vi "图形化显示数据-1.vi"() -> ()   [LabVIEW 2023]
panel:
  out "Waveform Graph 3":dbl[](graph)
  out "Waveform Chart 3":dbl(graph)
  out "Waveform Graph 2":dbl[](graph)
  out "Waveform Chart 2":dbl(graph)
  out "Waveform Graph":dbl[](graph)
  out "Waveform Chart":dbl(graph)
  # "图形化显示数据"
  # "极坐标系 Polar coordinates 是一种二维坐标系，它使用一个点到原点的距离（称为极径）和该点与正x轴之间的夹角（称为极角）来表示一个点的坐标。"
  # "(r, θ) r 是 极径 点到原点的距离， θ 是 点到 x轴 的 夹脚， 通常 极坐标 用来处理 正数。"
  # "LabVIEW 中最常见的曲线格式是在一个直角坐标系中用 X 轴表示时间，Y 轴表示数据值。"
  # "分析数据走向趋势"
  # "Chart 会保存以前的数据，因为有缓存区， graph 没有缓存区，每次清空"
  # "chart 的属性节点 选择历史，然后双击历史节点属性 选择 改变输出 为输入"
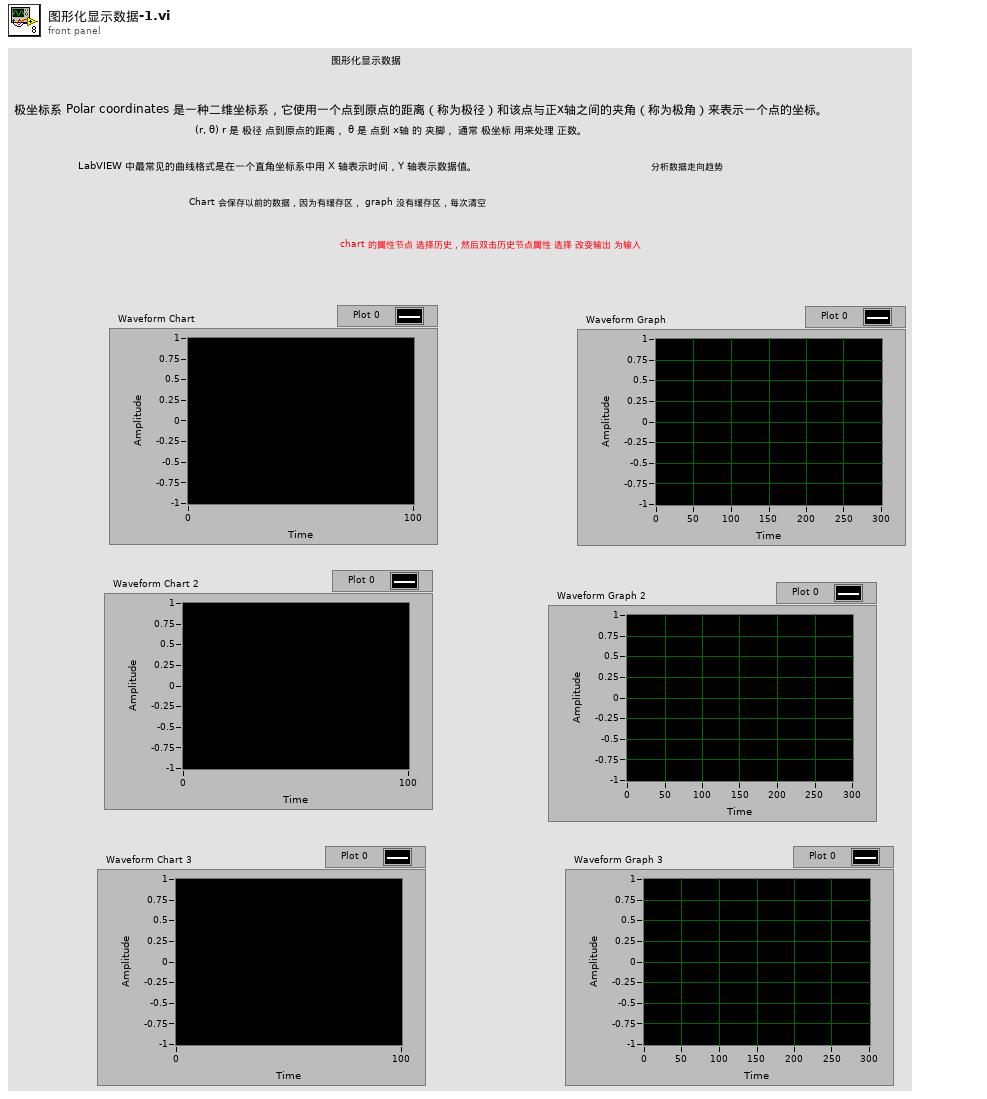
[diagram p1: front panel]
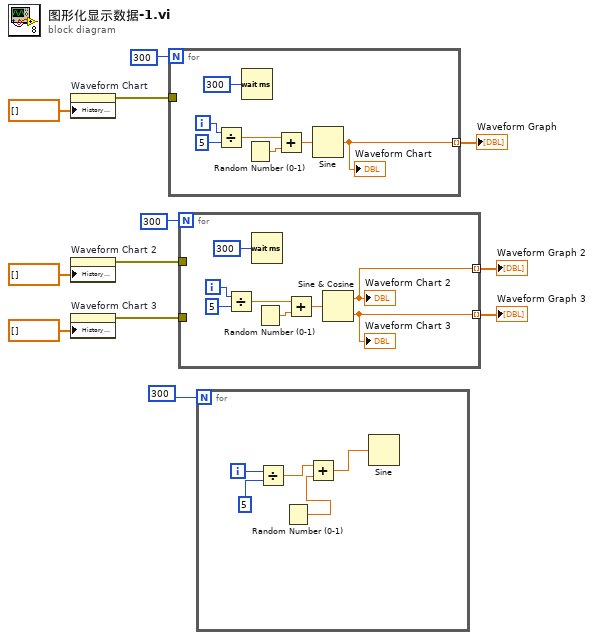
[diagram p0: block diagram]
diagram:
  n1 = property on="Waveform Chart" class="WFChart (strict)"("History Data"=dbl[] []) -> (error out=w6:errorcluster)  [unwired: 2 in, 1 out]
  n2 = property on="Waveform Chart 2" class="WFChart (strict)"("History Data"=dbl[] []) -> (error out=w2:errorcluster)  [unwired: 2 in, 1 out]
  n3 = property on="Waveform Chart 3" class="WFChart (strict)"("History Data"=dbl[] []) -> (error out=w4:errorcluster)  [unwired: 2 in, 1 out]
  n4 = for {
    N: 300 -> [_]
    tunnel: [w13] -> w11 mode=indexing
    tunnel: w6 -> [_]
    i -> [w19]
    n5 = Divide(x=w19, y=5) -> (x/y=w17:dbl)
    n6 = Wait (ms)(milliseconds to wait=u32 300) -> ()  [unwired: 1 out]
    n7 = Random Number (0-1)() -> (number: 0 to 1=w16:dbl)
    n8 = Add(x=w17, y=w16) -> (x+y=w15:dbl)
    n9 = Sine(x=w15) -> (sin(x)=w13:dbl)
    "Waveform Chart" <- w13
  }
  "Waveform Graph" <- w11
  n10 = for {
    N: 300 -> [_]
    tunnel: [w21] -> w9 mode=indexing
    tunnel: [w20] -> w8 mode=indexing
    tunnel: w4 -> [_]
    tunnel: w2 -> [_]
    i -> [w27]
    n11 = Divide(x=w27, y=5) -> (x/y=w25:dbl)
    n12 = Wait (ms)(milliseconds to wait=u32 300) -> ()  [unwired: 1 out]
    n13 = Random Number (0-1)() -> (number: 0 to 1=w24:dbl)
    n14 = Add(x=w25, y=w24) -> (x+y=w22:dbl)
    n15 = Sine & Cosine(0:w22) -> (1:w21:dbl, 2:w20:dbl)
    "Waveform Chart 2" <- w21
    "Waveform Chart 3" <- w20
  }
  "Waveform Graph 2" <- w9
  "Waveform Graph 3" <- w8
  n16 = for {
    N: 300 -> [_]
    i -> [w32]
    n17 = Divide(x=w32, y=5) -> (x/y=w30:dbl)
    n18 = Random Number (0-1)() -> (number: 0 to 1=w29:dbl)
    n19 = Add(x=w30, y=w29) -> (x+y=w28:dbl)
    n20 = Sine(x=w28) -> ()  [unwired: 1 out]
  }
